vi "Pendant.vi"() -> ()   [LabVIEW 2013]
uses:
  ROS/Code/SubVIs/BaxterSide.ctl
  <vilib>/Analysis/Matrix/Datatypes/RealMatrix.ctl
  ROS/Code/Console/Servers/ServerSubs/(nist) Arm Globals.vi
  Arm Globals.vi
  Prim/Fwd Kenimatics - array.vi
  Move/Move Axis.vi
  <vilib>/Utility/config.llb/Read Key (String).vi
  <vilib>/Utility/config.llb/Write Key (String).vi
  <vilib>/Utility/config.llb/NI_LVConfig.lvlib
  <vilib>/Analysis/Matrix/NI_Matrix.lvlib
panel:
  in  "R:End":bool
  in  "R:Pause":bool
  out "T":T1=[[0.016284994521607307, 0.9998576764567041, 0.0044074691186384496, -12.095922523672678], [0.9998670931969393, -0.01628143110047913, -0.0008431744914288715, -1019.3924117975101], [-0.0007712945830650122, 0.004420614427981981, -0.999989931585686, 240.25900755427352], [0.0, 0.0, 0.0, 1.0]] format="%.3f"
  in  "Mode":enum32{"Slew", "Shift", "Set", "Save", "Manual"}(tab)
  in  "mm":dbl(knob) scale=0.0..50.0
  in  "Value":dbl
  in  "Show":bool
  in  "Load":bool
  in  "Save":bool
  in  "section":string
  in  "name":string
  in  "Joints":dbl[](array[numeric])=[-40.0, -65.0, 0.0, 90.0, 0.0, 65.0, 0.0] format="%.1f"
  in  "Safe":bool
  in  "Gripper":bool
  in  "Side":T2=enum."right"
  in  "Make Vertical":bool
  in  "Speed":dbl(knob) caption="mm/s" scale=0.0..200.0
  out "+A":bool
  out "-Z":bool
  out "-A":bool
  out "+Z":bool
  out "String":string
  in  "end":bool
  out "+Y":bool
  out "-X":bool
  out "-Y":bool
  out "+X":bool
  # "Uses the \"Positions.cfg\" file."
  # "Push 4 wrist buttons\nto move arm.\nChange mode when done."
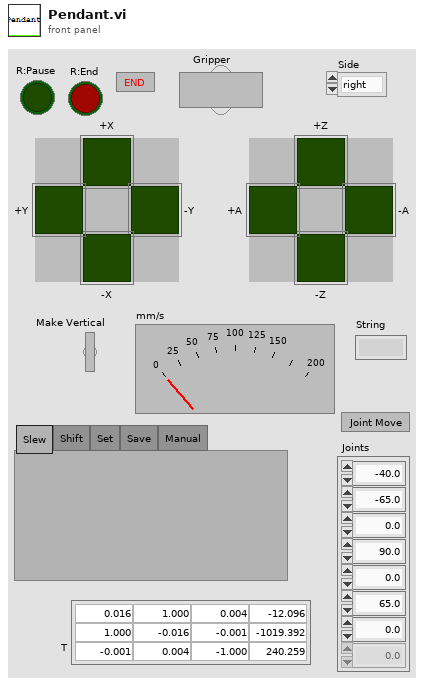
[diagram p1: front panel]
types:
  T1 = typedef "NI_Matrix.lvlib/RealMatrix.ctl" = dbl[][]
  T2 = typedef "BaxterSide.ctl" = enum16{"left", "right"}
  T3 = cluster{"X":dbl, "Y":dbl, "Z":dbl, "O":dbl, "A":dbl, "T":dbl}
  T4 = cluster{"Value":dbl, "Value":dbl, "Value":dbl, dbl, dbl, dbl}
  T5 = typedef "NI_LVConfig.lvlib/Config Data RefNum.ctl" = refnum<k1>
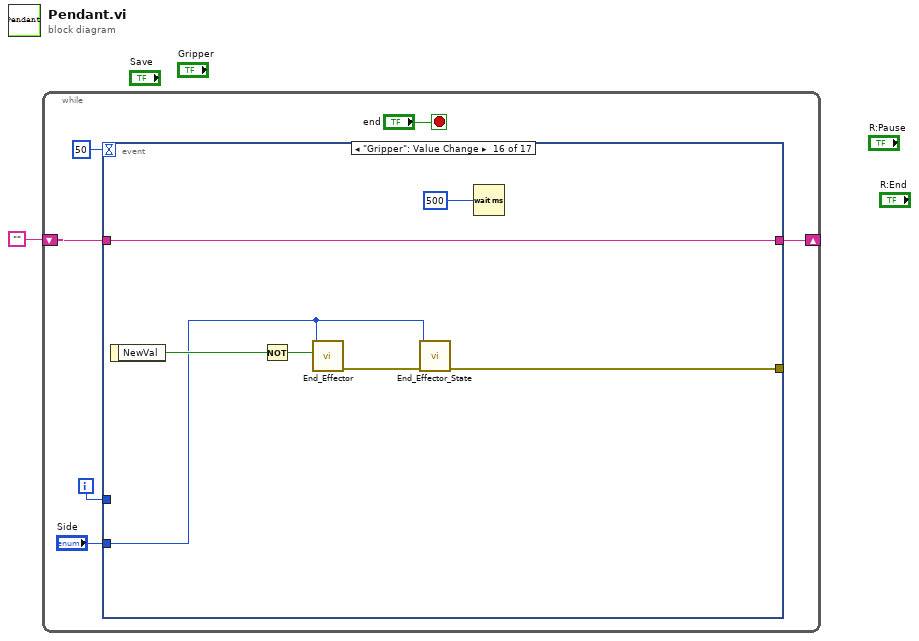
[diagram p0: block diagram]
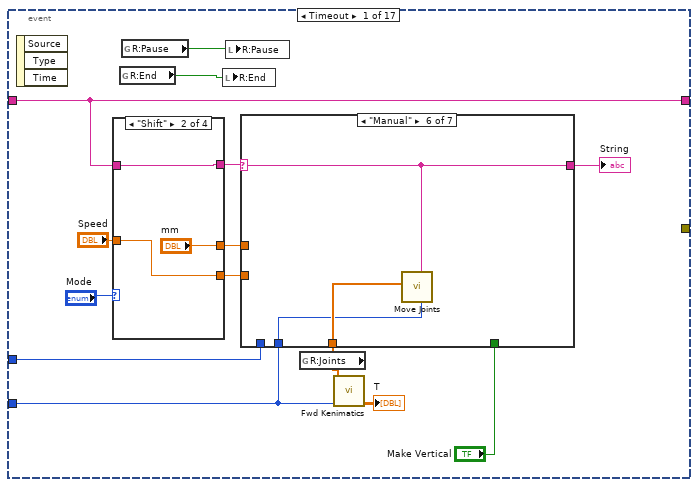
[diagram p2: hidden frame]
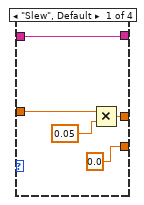
[diagram p3: hidden frame]
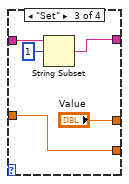
[diagram p4: hidden frame]
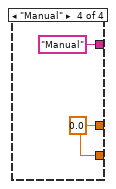
[diagram p5: hidden frame]
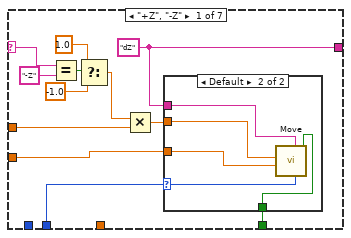
[diagram p6: hidden frame]
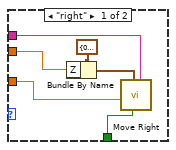
[diagram p7: hidden frame]
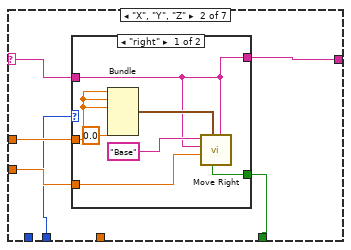
[diagram p8: hidden frame]
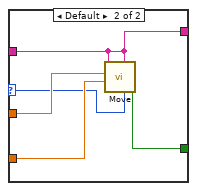
[diagram p9: hidden frame]
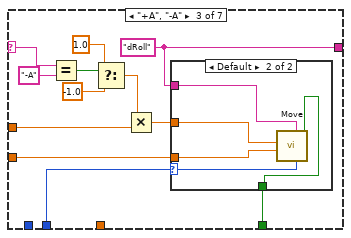
[diagram p10: hidden frame]
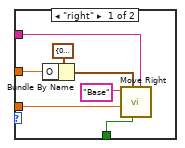
[diagram p11: hidden frame]
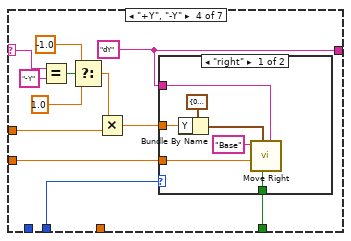
[diagram p12: hidden frame]
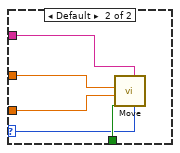
[diagram p13: hidden frame]
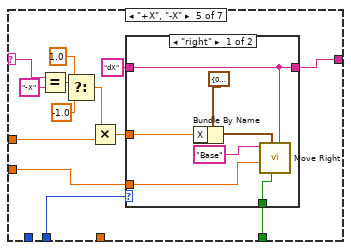
[diagram p14: hidden frame]
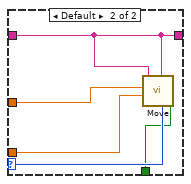
[diagram p15: hidden frame]
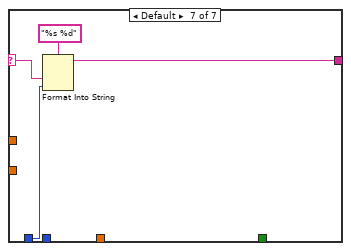
[diagram p16: hidden frame]
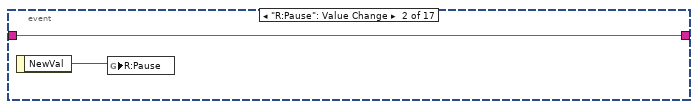
[diagram p17: hidden frame]
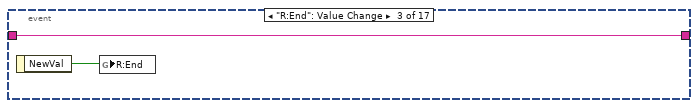
[diagram p18: hidden frame]
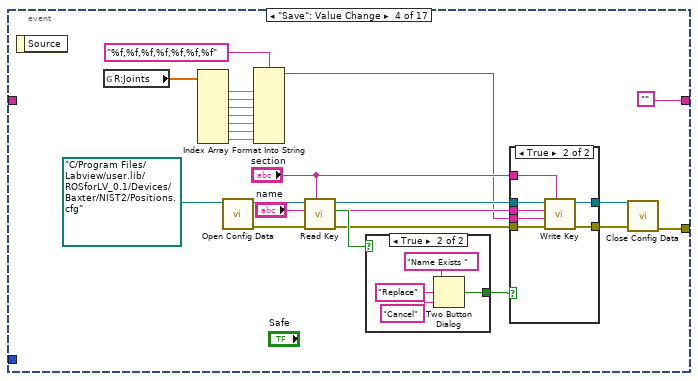
[diagram p19: hidden frame]
diagram:
  n1 = while {
    shift-right: [w4] -> _
    shift-left: "" -> [w3]
    i -> [w5]
    stop <- "end" stop-if-true
    n2 = event shown="[15] \"Gripper\": Value Change" {
      selector: _ -> [_ _ _ _ _ _ _ _ _ _ _ _ _ _ _ _ _]
      dyn-events: _ -> [_ _ _ _ _ _ _ _ _ _ _ _ _ _ _ _ _]
      timeout: 50 -> [_ _ _ _ _ _ _ _ _ _ _ _ _ _ _ _ _]
      tunnel: w5 -> [w21 _ _ _ _ _ _ _ _ _ _ _ _ _ _ _ _]
      tunnel: [w15 w158 w160 "" "" _ "+X" ("String") "" "-Y" ("String") "+Z" ("String") "-Z" ("String") "-A" ("String") "+A" ("String") "-X" ("String") "+Y" ("String") w245 ""] -> w4
      tunnel: w3 -> [w15 w158 w160 _ _ _ _ _ _ _ _ _ _ _ _ w245 _]
      tunnel: "Side" -> [w12 _ _ _ _ _ _ _ _ _ _ _ _ _ _ w246 w254]
      tunnel: [_ _ _ w172 w209 _ _ _ _ _ _ _ _ _ _ w244 _] -> _
      event Timeout {
        n3 = event-data() -> ()  [unwired: 1 in, 3 out]
        n4 = case shown="\"Shift\"" "Mode" {
          tunnel: "Speed" -> [w25 w28 w33 _]
          tunnel: [w24 "mm" "Value" w36] -> w18
          tunnel: [0.0 ("Speed") w28 w33 w36] -> w17
          tunnel: w15 -> [w22 w27 w32 _]
          tunnel: [w22 w27 w30 "Manual"] -> w14
          frame "Slew", Default {
            n5 = Multiply(x=w25, y=0.05) -> (x*y=w24:dbl)
          }
          frame "Shift" {
          }
          frame "Set" {
            n6 = String Subset(string=w32, offset (0)=1) -> (substring=w30:string)  [unwired: 1 in]
          }
          frame "Manual" {
            w36 = 0.0 ("Value")
          }
        }
        n7 = global read "Arm Globals.vi" "R:End"() -> (w10:bool)
        n8 = global read "Arm Globals.vi" "R:Pause"() -> (w11:bool)
        n9 = local write "R:End"(w10) -> ()
        n10 = local write "R:Pause"(w11) -> ()
        n11 = global read "(nist) Arm Globals.vi" "R:Joints"() -> (w8:dbl[])
        n12 = case shown="\"Manual\"" w14 {
          selector: w14 -> [w48 w60 w89 w113 w138 w152 w155]
          tunnel: w21 -> [_ _ _ _ _ _ w156]
          tunnel: [w39 w61 w83 w103 w127 w152 w154] -> w9
          tunnel: w18 -> [w44 w65 w79 w109 w133 _ _]
          tunnel: w12 -> [w38 w63 w82 w105 w129 w151 _]
          tunnel: "Make Vertical" -> [w37 w62 w78 w102 w126 _ _]
          tunnel: w17 -> [w41 w64 w81 w106 w130 _ _]
          tunnel: w8 -> [_ _ _ _ _ w153 _]
          frame "+Z", "-Z" {
            w39 = "dZ"
            n13 = Equal?(x=w48, y="-Z") -> (x = y?=w46:bool)
            n14 = Select(t=1.0, s=w46, f=-1.0) -> (s? t:f=w43:dbl)
            n15 = Multiply(x=w43, y=w44) -> (x*y=w40:dbl)
            n16 = case shown="Default" w38 {
              selector: w38 -> [_ w56]
              tunnel: w40 -> [w52 w59]
              tunnel: w41 -> [w50 w58]
              tunnel: w39 -> [w53 w57]
              tunnel: w37 -> [w49 w55]
              frame "right" {
                n17 = Bundle By Name(cluster=T3 {"X"=0.0, "Y"=0.0, "Z"=0.0, "O"=0.0, "A"=0.0, "T"=0.0} ("Goal Axes"), "Z"=w52) -> (w51:T3)
                n18 = call "Move Right.vi"("Label"=w53, "Make Vertical"=w49, "Goal"=w51, "Speed"=w50) -> ()  [unwired: 3 in, 5 out]
              }
              frame Default {
                n19 = call-poly "Move.vi"("Make Vertical"=w55, "Side"=w56, "Label"=w57, "Speed"=w58, "Value"=w59, "Location"=w57) -> ()  [unwired: 5 in, 1 out]
              }
            }
          }
          frame "X", "Y", "Z" {
            n20 = case shown="\"right\"" w63 {
              selector: w63 -> [_ w75]
              tunnel: w65 -> [w72 w77]
              tunnel: w60 -> [w66 w73]
              tunnel: w64 -> [w67 w76]
              tunnel: w62 -> [w68 w74]
              tunnel: [w66 w73] -> w61
              frame "right" {
                w71 = 0.0
                n21 = Bundle("Value"=w72, "Value"=w72, "Value"=w72, w71, w71, w71) -> (w70:T4)  [unwired: 1 in]
                n22 = call "Move Right.vi"("Label"=w66, "Make Vertical"=w68, "Goal"=w70, "Speed"=w67, "Mask"=w66, "Location"="Base") -> ()  [unwired: 1 in, 5 out]
              }
              frame Default {
                n23 = call-poly "Move.vi"("Make Vertical"=w74, "Side"=w75, "Label"=w73, "Speed"=w76, "Value"=w77, "Location"=w73) -> ()  [unwired: 5 in, 1 out]
              }
            }
          }
          frame "+A", "-A" {
            w83 = "dRoll"
            n24 = Equal?(x=w89, y="-A") -> (x = y?=w87:bool)
            n25 = Select(t=1.0, s=w87, f=-1.0) -> (s? t:f=w85:dbl)
            n26 = Multiply(x=w85, y=w79) -> (x*y=w80:dbl)
            n27 = case shown="Default" w82 {
              selector: w82 -> [_ w98]
              tunnel: w80 -> [w94 w101]
              tunnel: w81 -> [w91 w100]
              tunnel: w83 -> [w95 w99]
              tunnel: w78 -> [w90 w97]
              frame "right" {
                n28 = Bundle By Name(cluster=T3 {"X"=0.0, "Y"=0.0, "Z"=0.0, "O"=0.0, "A"=0.0, "T"=0.0} ("Goal Axes"), "O"=w94) -> (w92:T3)
                n29 = call "Move Right.vi"("Label"=w95, "Make Vertical"=w90, "Goal"=w92, "Speed"=w91, "Location"="Base") -> ()  [unwired: 2 in, 5 out]
              }
              frame Default {
                n30 = call-poly "Move.vi"("Make Vertical"=w97, "Side"=w98, "Label"=w99, "Speed"=w100, "Value"=w101, "Location"=w99) -> ()  [unwired: 5 in, 1 out]
              }
            }
          }
          frame "+Y", "-Y" {
            w103 = "dY"
            n31 = Equal?(x=w113, y="-Y") -> (x = y?=w111:bool)
            n32 = Select(t=-1.0, s=w111, f=1.0) -> (s? t:f=w108:dbl)
            n33 = Multiply(x=w108, y=w109) -> (x*y=w104:dbl)
            n34 = case shown="\"right\"" w105 {
              selector: w105 -> [_ w121]
              tunnel: w104 -> [w118 w125]
              tunnel: w102 -> [w115 w124]
              tunnel: w106 -> [w114 w123]
              tunnel: w103 -> [w119 w122]
              frame "right" {
                n35 = Bundle By Name(cluster=T3 {"X"=0.0, "Y"=0.0, "Z"=0.0, "O"=0.0, "A"=0.0, "T"=0.0} ("Goal Axes"), "Y"=w118) -> (w117:T3)
                n36 = call "Move Right.vi"("Label"=w119, "Make Vertical"=w115, "Goal"=w117, "Speed"=w114, "Location"="Base") -> ()  [unwired: 2 in, 5 out]
              }
              frame Default {
                n37 = call-poly "Move.vi"("Make Vertical"=w124, "Side"=w121, "Label"=w122, "Speed"=w123, "Value"=w125, "Location"=w122) -> ()  [unwired: 5 in, 1 out]
              }
            }
          }
          frame "+X", "-X" {
            n38 = Equal?(x=w138, y="-X") -> (x = y?=w136:bool)
            n39 = Select(t=1.0, s=w136, f=-1.0) -> (s? t:f=w132:dbl)
            n40 = Multiply(x=w132, y=w133) -> (x*y=w134:dbl)
            n41 = case shown="\"right\"" w129 {
              selector: w129 -> [_ w148]
              tunnel: [w143 w146] -> w127
              tunnel: w134 -> [w144 w150]
              tunnel: w126 -> [w140 w147]
              tunnel: w130 -> [w139 w149]
              tunnel: "dX" -> [w143 w146]
              frame "right" {
                n42 = Bundle By Name(cluster=T3 {"X"=0.0, "Y"=0.0, "Z"=0.0, "O"=0.0, "A"=0.0, "T"=0.0} ("Goal Axes"), "X"=w144) -> (w142:T3)
                n43 = call "Move Right.vi"("Label"=w143, "Make Vertical"=w140, "Goal"=w142, "Speed"=w139, "Location"="Base") -> ()  [unwired: 2 in, 5 out]
              }
              frame Default {
                n44 = call-poly "Move.vi"("Make Vertical"=w147, "Side"=w148, "Label"=w146, "Speed"=w149, "Value"=w150, "Location"=w146) -> ()  [unwired: 5 in, 1 out]
              }
            }
          }
          frame "Manual" {
            n45 = call "Move Joints.vi"("Side"=w151, "Label"=w152, "Goal"=w153) -> ()  [unwired: 7 in, 2 out]
          }
          frame Default {
            n46 = Format Into String(format string="%s %d", w155, w156) -> (resulting string=w154:string)  [unwired: 2 in, 1 out]
          }
        }
        "String" <- w9
        n47 = call-poly "Fwd Kenimatics.vi"("Side"=w12, "Joints"=w8) -> ("Matrix"=→"T":T1)  [unwired: 8 in, 1 out]
      }
      event "R:Pause": Value Change {
        n48 = event-data() -> ("NewVal"=w159:bool)  [unwired: 1 in]
        n49 = global write "Arm Globals.vi" "R:Pause"(w159) -> ()
      }
      event "R:End": Value Change {
        n50 = event-data() -> ("NewVal"=w161:bool)  [unwired: 1 in]
        n51 = global write "Arm Globals.vi" "R:End"(w161) -> ()
      }
      event "Save": Value Change {
        n52 = event-data() -> ()  [unwired: 1 in, 1 out]
        n53 = global read "(nist) Arm Globals.vi" "R:Joints"() -> (w182:dbl[])
        n54 = Index Array(array=w182) -> (element #1=w183:dbl, element #2=w181:dbl, element #3=w180:dbl, element #4=w179:dbl, element #5=w178:dbl, element #6=w177:dbl, element #7=w176:dbl)  [unwired: 7 in]
        n55 = call <vilib>:"Open Config Data.vi"("configuration file path"=path "C:/Program Files/Labview/user.lib/ROSforLV_0.1/Devices/Baxter/NIST2/Positions.cfg") -> ("error out"=w170:errorcluster, "refnum"=w171:T5)  [unwired: 8 in, 1 out]
        n56 = Format Into String(format string="%f,%f,%f,%f,%f,%f,%f", w183, w181, w180, w179, w178, w177, w176) -> (resulting string=w163:string)  [unwired: 2 in, 1 out]
        n57 = call-poly <vilib>:"Read Key.vi"("section"="section", "error in (no error)"=w170, "key"="name", "refnum"=w171) -> ("error out"=w166:errorcluster, "found?"=w169:bool, "refnum out"=w167:T5)  [unwired: 4 in, 1 out]
        n58 = case shown="True" w169 {
          tunnel: [TRUE ("T button?") w195] -> w168
          frame False {
          }
          frame True {
            n59 = Two Button Dialog(message="Name Exists ", 1:"Cancel" ("F button name (\"Cancel\")"), 2:"Replace" ("T button name (\"OK\")")) -> (T button?=w195:bool)
          }
        }
        n60 = case shown="True" w168 {
          tunnel: [w186 w193] -> w174
          tunnel: [w185 w192] -> w173
          tunnel: w167 -> [w186 w191]
          tunnel: w166 -> [w185 w190]
          tunnel: "section" -> [_ w189]
          tunnel: "name" -> [_ w188]
          tunnel: w163 -> [_ w187]
          frame False {
          }
          frame True {
            n61 = call-poly <vilib>:"Write Key.vi"("section"=w189, "error in (no error)"=w190, "value"=w187, "key"=w188, "refnum"=w191) -> ("error out"=w192:errorcluster, "refnum out"=w193:T5)  [unwired: 4 in, 1 out]
          }
        }
        n62 = call <vilib>:"Close Config Data.vi"("error in (no error)"=w173, "refnum"=w174) -> ("error out"=w172:errorcluster)  [unwired: 8 in, 1 out]
      }
      event "Load": Value Change {
        n63 = event-data() -> ()  [unwired: 1 in, 1 out]
        n64 = local read "section"() -> (w204:string)
        n65 = local read "name"() -> (w203:string)
        n66 = call <vilib>:"Open Config Data.vi"("configuration file path"=path "C:/Program Files/Labview/user.lib/ROSforLV_0.1/Devices/Baxter/NIST2/Positions.cfg") -> ("error out"=w207:errorcluster, "refnum"=w208:T5)  [unwired: 8 in, 1 out]
        n67 = call-poly <vilib>:"Read Key.vi"("section"=w204, "error in (no error)"=w207, "key"=w203, "refnum"=w208) -> ("error out"=w201:errorcluster, "value"=w200:string, "found?"=w206:bool, "refnum out"=w202:T5)  [unwired: 4 in]
        n68 = case shown="False" w206 {
          tunnel: [FALSE ("T button?") TRUE ("T button?")] -> w205
          frame False {
            n69 = One Button Dialog(message="Name Does Not Exist ") -> ()  [unwired: 1 in, 1 out]
          }
          frame True {
          }
        }
        n70 = call <vilib>:"Close Config Data.vi"("error in (no error)"=w201, "refnum"=w202) -> ("error out"=w209:errorcluster)  [unwired: 8 in, 1 out]
        n71 = case shown="True" w205 {
          tunnel: w200 -> [_ w220]
          frame False {
          }
          frame True {
            n72 = Scan From String(format string="%f,%f,%f,%f,%f,%f,%f", input string=w220) -> (output 1=w218:dbl, output 2=w217:dbl, output 3=w216:dbl, output 4=w215:dbl, output 5=w214:dbl, output 6=w213:dbl, output 7=w212:dbl)  [unwired: 9 in, 3 out]
            n73 = Build Array(w218, w217, w216, w215, w214, w213, w212) -> (w211:dbl[])
            n74 = local write "Joints"(w211) -> ()
          }
        }
      }
      event "Show": Value Change {
        n75 = event-data() -> ()  [unwired: 1 in, 6 out]
        n76 = call "Pendant, show poses.vi"() -> ("position"=w224:string, "group"=w225:string)  [unwired: 8 in]
        n77 = local write "name"(w224) -> ()
        n78 = local write "section"(w225) -> ()
      }
      event "+X": Mouse Down {
        n79 = event-data() -> ()  [unwired: 1 in, 1 out]
        n80 = local write "+X"(TRUE ("+X")) -> ()
      }
      event "+X", "-Y", "-X", "+Y", "+Z", "-A", "-Z", "+A": Mouse Leave; "+X", "-Y", "-X", "+Y", "+Z", "-A", "-Z", "+A": Mouse Up {
        w228 = FALSE ("+X")
        n81 = event-data() -> ()  [unwired: 1 in, 3 out]
        "-X" <- w228
        "-Y" <- w228
        "+Y" <- w228
        "+X" <- w228
        "+Z" <- w228
        "-Z" <- w228
        "+A" <- w228
        "-A" <- w228
      }
      event "-Y": Mouse Down {
        n82 = event-data() -> ()  [unwired: 1 in, 3 out]
        n83 = local write "-Y"(TRUE ("-Y")) -> ()
      }
      event "+Z": Mouse Down {
        n84 = event-data() -> ()  [unwired: 1 in, 3 out]
        n85 = local write "+Z"(TRUE ("-Y")) -> ()
      }
      event "-Z": Mouse Down {
        n86 = event-data() -> ()  [unwired: 1 in, 3 out]
        n87 = local write "-Z"(TRUE ("-Y")) -> ()
      }
      event "-A": Mouse Down {
        n88 = event-data() -> ()  [unwired: 1 in, 3 out]
        n89 = local write "-A"(TRUE ("-Y")) -> ()
      }
      event "+A": Mouse Down {
        n90 = event-data() -> ()  [unwired: 1 in, 3 out]
        n91 = local write "+A"(TRUE ("-Y")) -> ()
      }
      event "-X": Mouse Down {
        n92 = event-data() -> ()  [unwired: 1 in, 3 out]
        n93 = local write "-X"(TRUE) -> ()
      }
      event "+Y": Mouse Down? {
        n94 = event-data() -> ()  [unwired: 1 in, 3 out]
        n95 = local write "+Y"(TRUE ("+Y")) -> ()
        n96 = event-data() -> ()  [unwired: 2 in, 1 out]
      }
      event "Gripper": Value Change {
        n97 = event-data() -> ("NewVal"=w247:bool)  [unwired: 1 in]
        n98 = Not(x=w247) -> (.not. x?=w248:bool)
        n99 = call "End_Effector.vi"("Close"=w248, "Side"=w246) -> ("error out"=w249:errorcluster)  [unwired: 6 in]
        n100 = call "End_Effector_State.vi"("error in"=w249, "Side"=w246) -> ("error out"=w244:errorcluster)  [unwired: 3 in, 3 out]
        n101 = Wait (ms)(milliseconds to wait=u32 500) -> ()  [unwired: 1 out]
      }
      event "Safe": Value Change {
        n102 = event-data() -> ()  [unwired: 1 in, 2 out]
        n103 = call "Move Joints.vi"("Side"=w254, "Label"="Safe", "Goal"="Joints") -> ("error out"=w253:errorcluster)  [unwired: 7 in, 1 out]
        n104 = flat-sequence {
          tunnel: [w257] -> _
          tunnel: w253 -> [w257]
          frame #0 {
            n105 = local write "Safe"(FALSE ("Safe")) -> ()
          }
        }
      }
    }
  }
